vi "TTA_Calibration_Routine.vi"() -> ()   [LabVIEW 2016]
uses:
  TTA_Controls/TTA_Control_Instrument_Cluster.ctl
  TTA_Globals/TTA_Instrument_Cluster.vi
  TTA_Globals/TTA_Global_Working_Directory.vi
  <vilib>/Utility/file.llb/Read Delimited Spreadsheet (string).vi
panel:
  out "Freq Array":T1(array[cluster])
  out "all rows":string[][](array[string])
  in  "Start":bool
  in  "WCS Template":path
  in  "IMT Template":path
  in  "Working Directory":path
  in  "AWS Template":path
  in  "DCS Template":path
  in  "PCS Template":path
  in  "Instrument Cluster":T2
  out "Calibration Status":string
  in  "error in":errorcluster
  out "2D Picture":picture
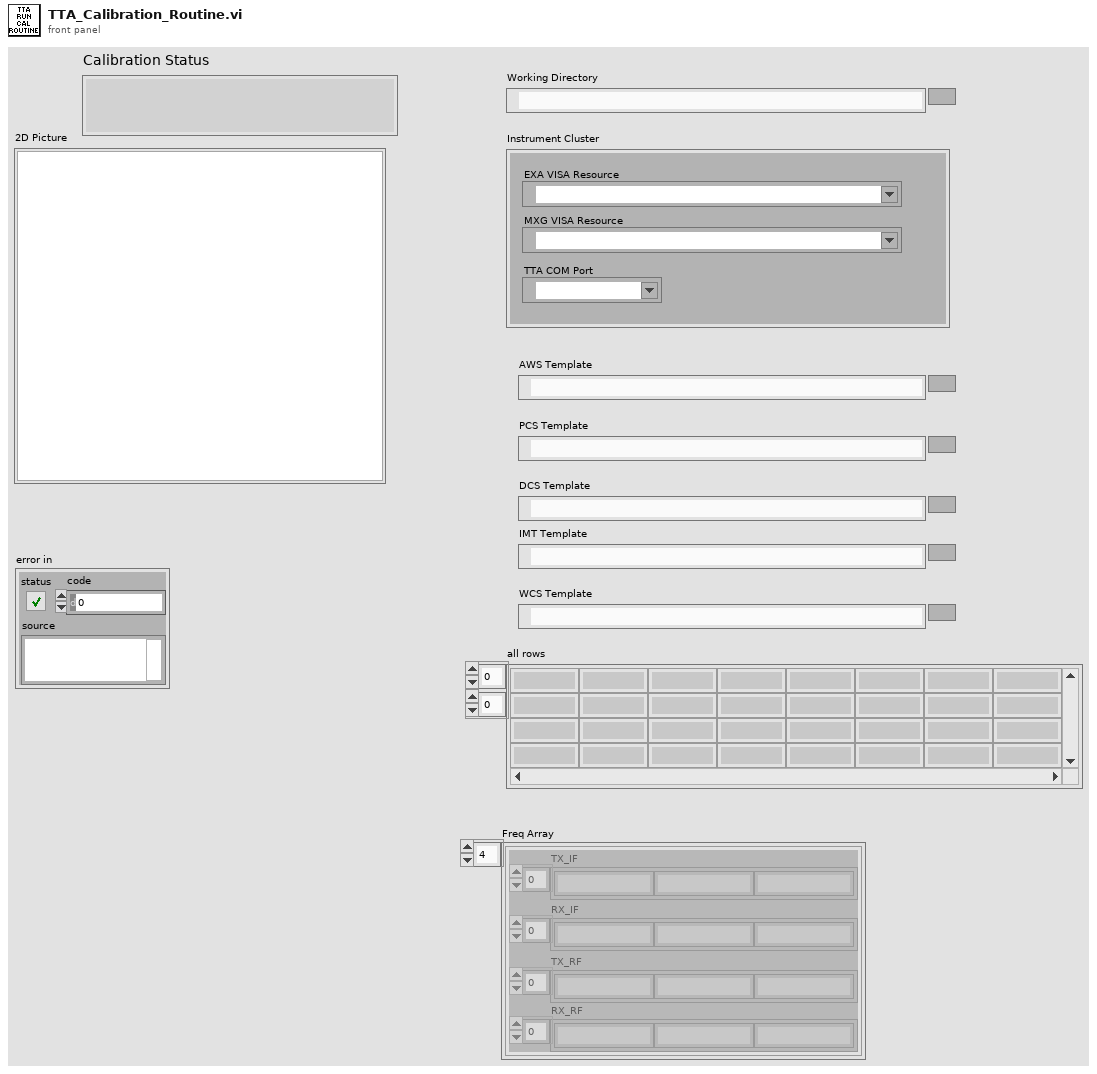
[diagram p1: front panel]
types:
  T1 = cluster{"TX_IF":string[], "RX_IF":string[], "TX_RF":string[], "RX_RF":string[]}[]
  T2 = typedef "TTA_Control_Instrument_Cluster.ctl" = cluster{"EXA VISA Resource":refnum<visa-resource-name>, "MXG VISA Resource":refnum<visa-resource-name>, "TTA COM Port":refnum<visa-resource-name>}
  T3 = cluster{"EXA VISA Resource":refnum<visa-resource-name>, "MXG VISA Resource":refnum<visa-resource-name>, "TTA COM Port":refnum<visa-resource-name>}
  T4 = cluster{"left":i16, "top":i16, "right":i16, "bottom":i16}
  T5 = cluster{"Width":u16, "Style":enum32{"Solid", "Dash", "Dot", "DashDot", "DashDotDot"}}
  T6 = enum16{"TX1", "TX2", "TX3", "TX4", "TXx3", "TXx4", "RX1", "RX2", "RX3", "RX4", "RXx3", "RXx4", "RFCal"}
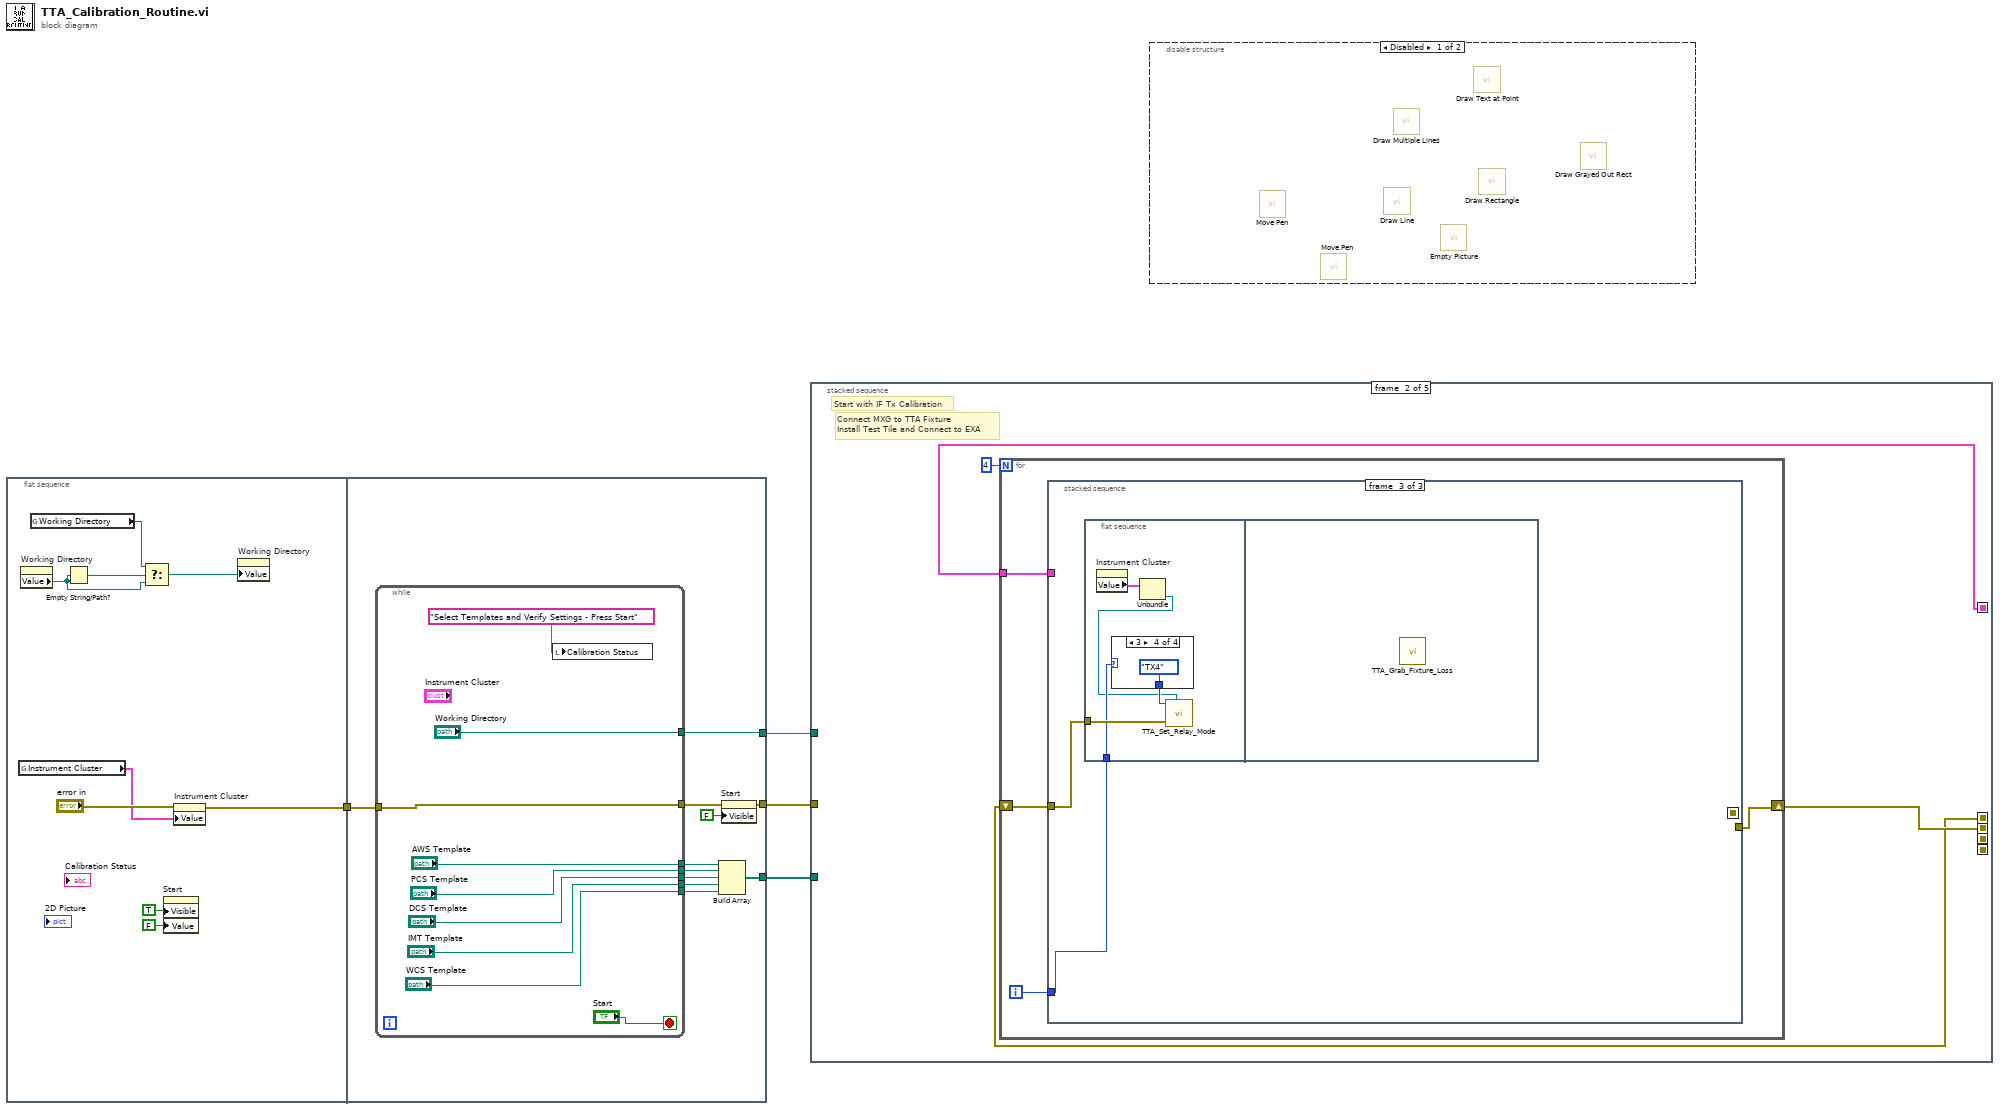
[diagram p0: block diagram]
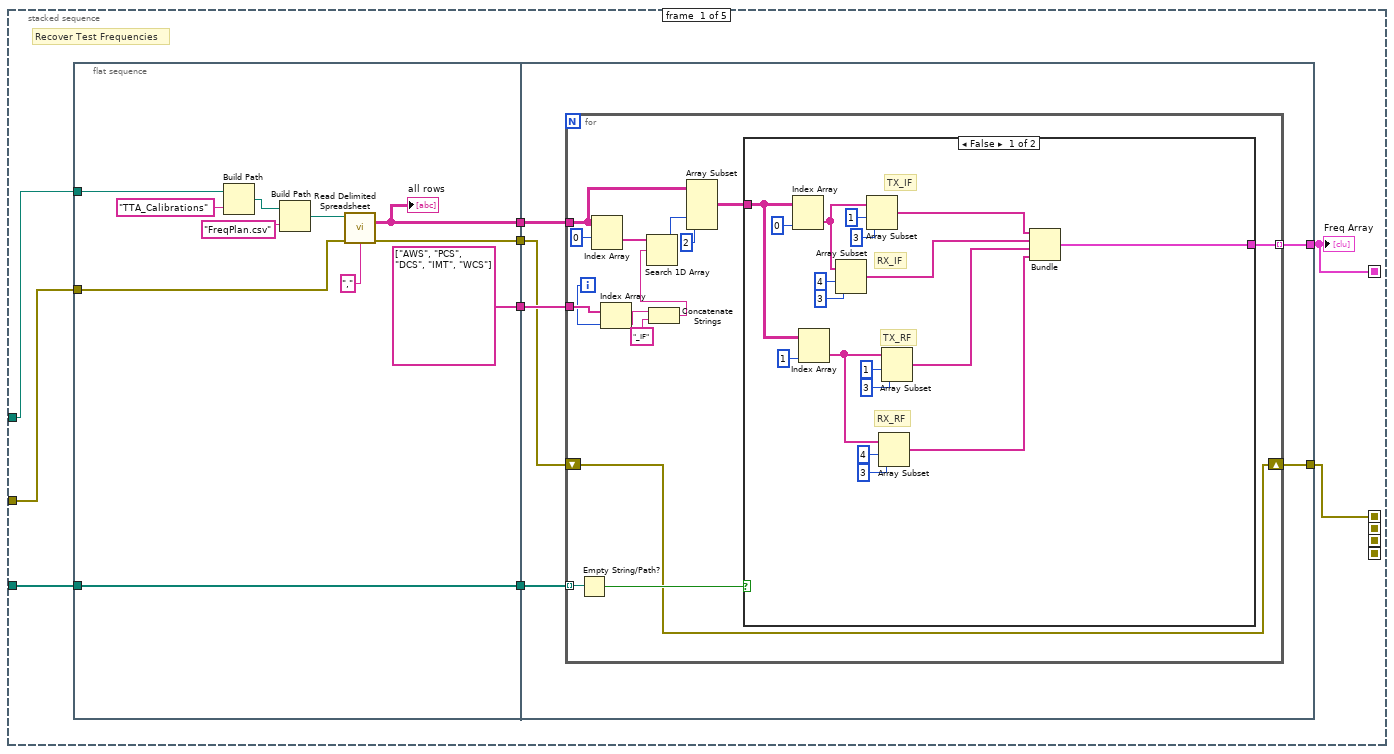
[diagram p3: hidden frame]
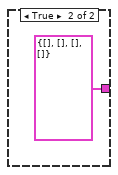
[diagram p4: hidden frame]
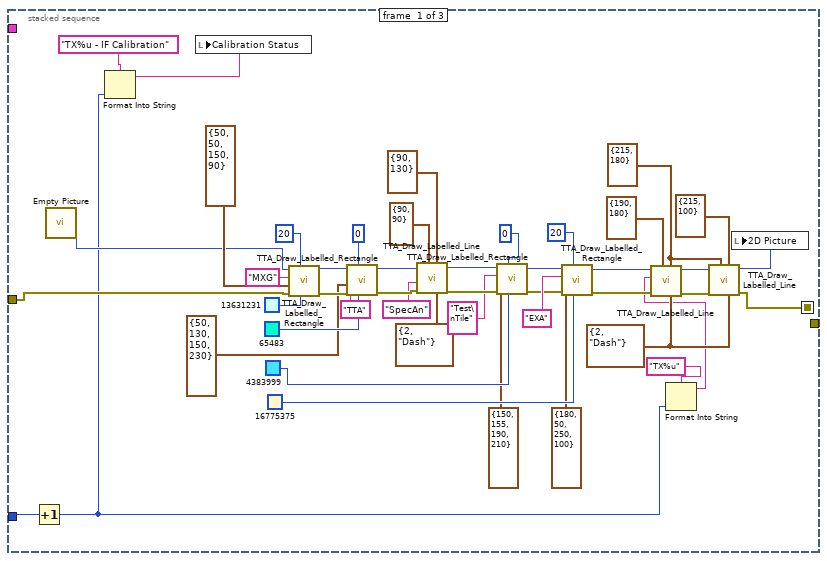
[diagram p5: hidden frame]
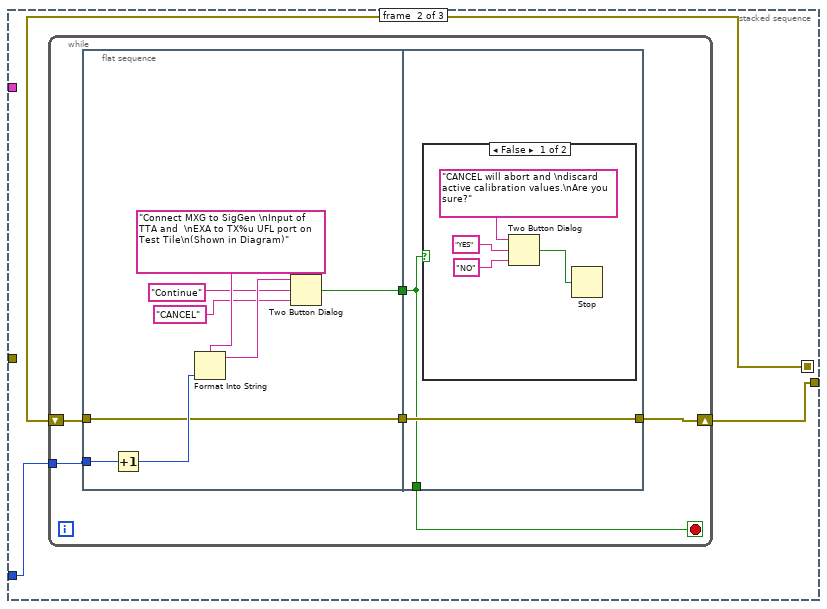
[diagram p6: hidden frame]
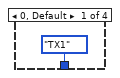
[diagram p8: hidden frame]
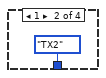
[diagram p9: hidden frame]
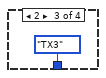
[diagram p10: hidden frame]
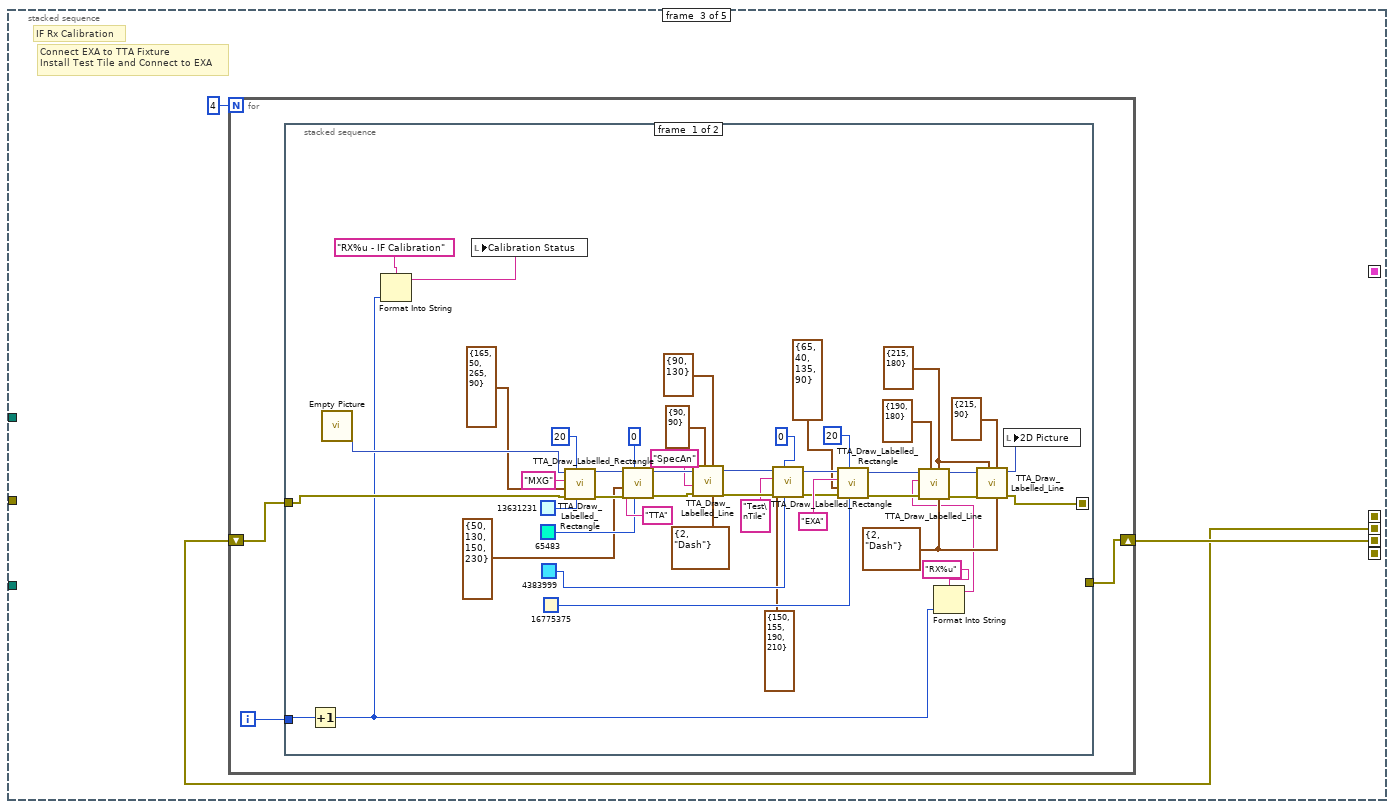
[diagram p11: hidden frame]
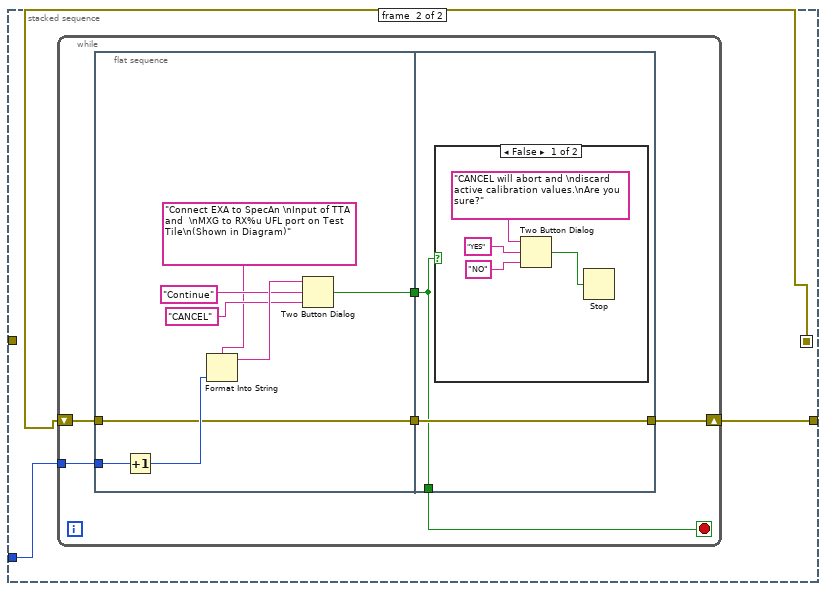
[diagram p12: hidden frame]
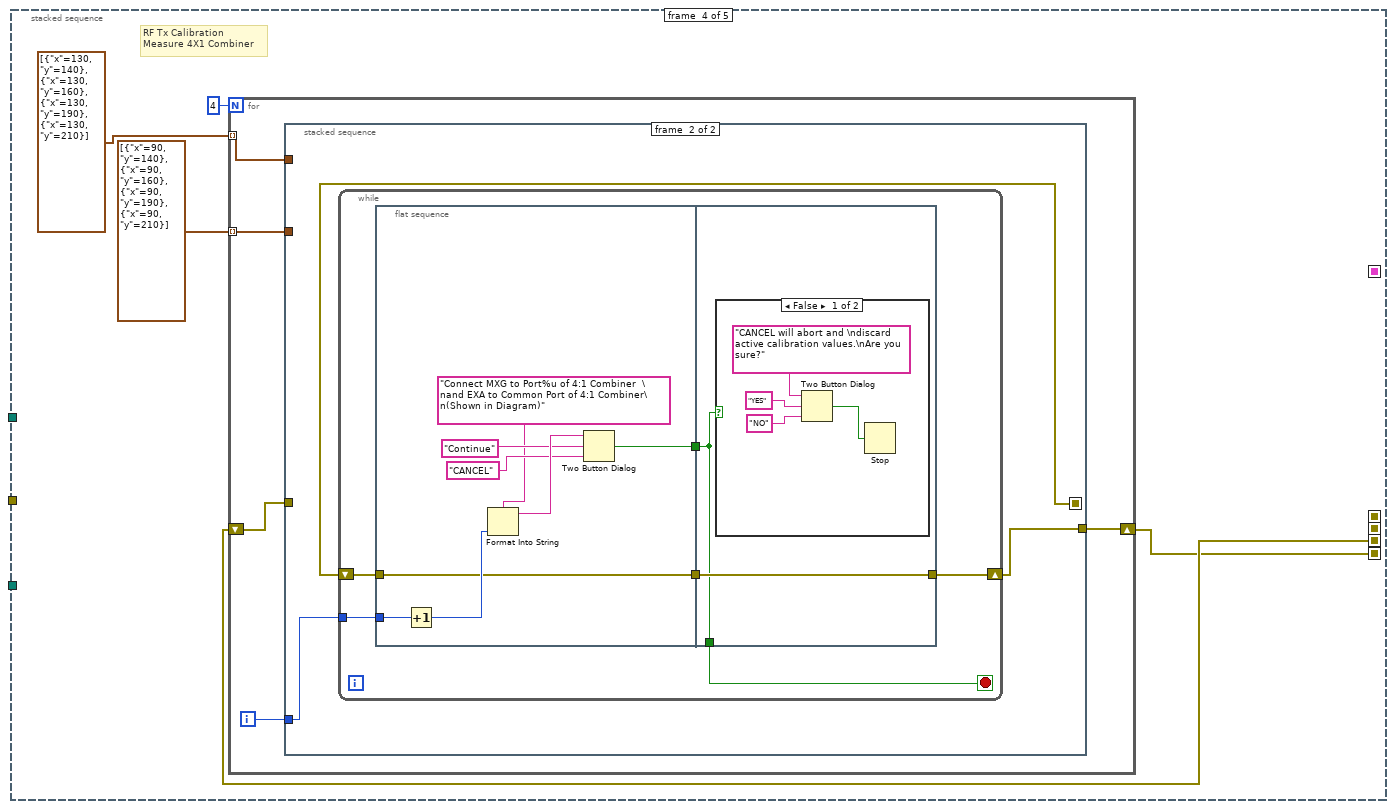
[diagram p14: hidden frame]
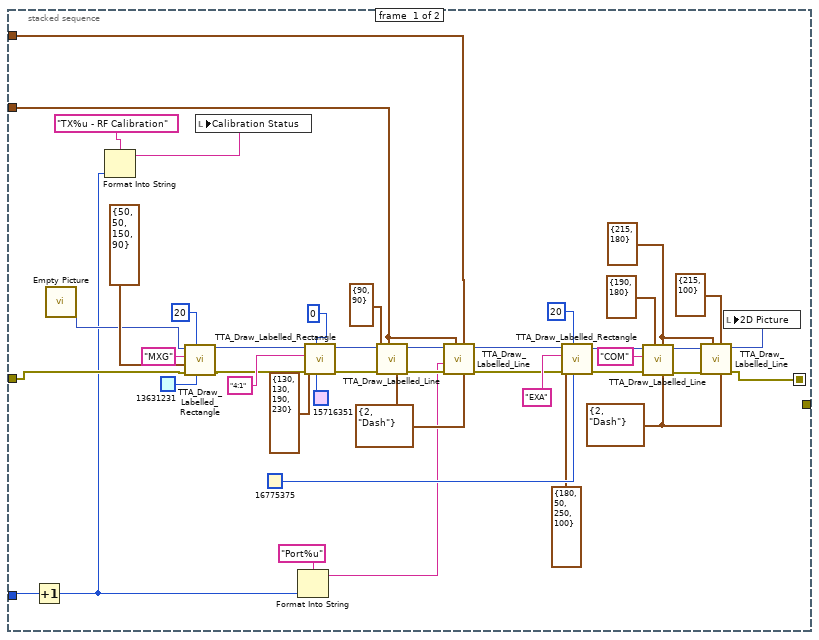
[diagram p15: hidden frame]
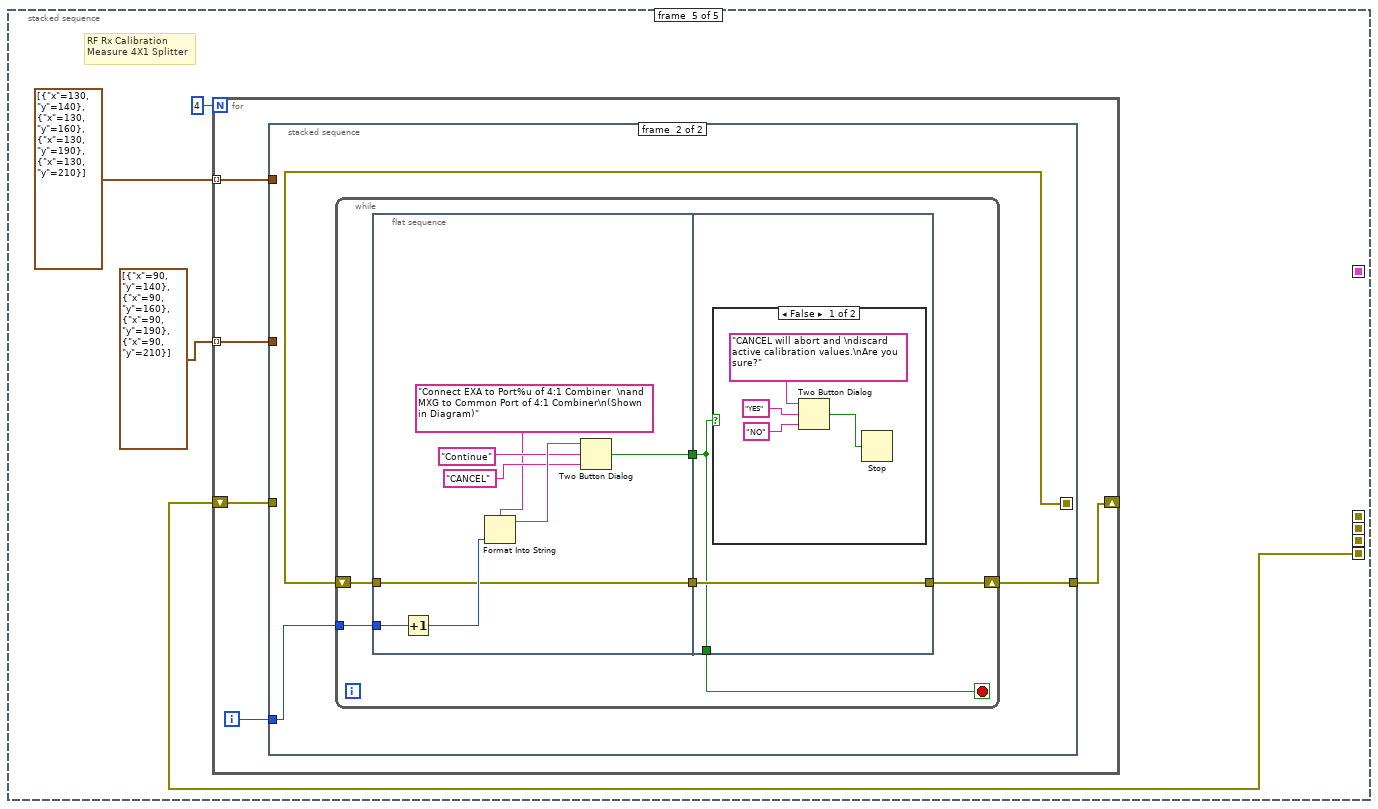
[diagram p17: hidden frame]
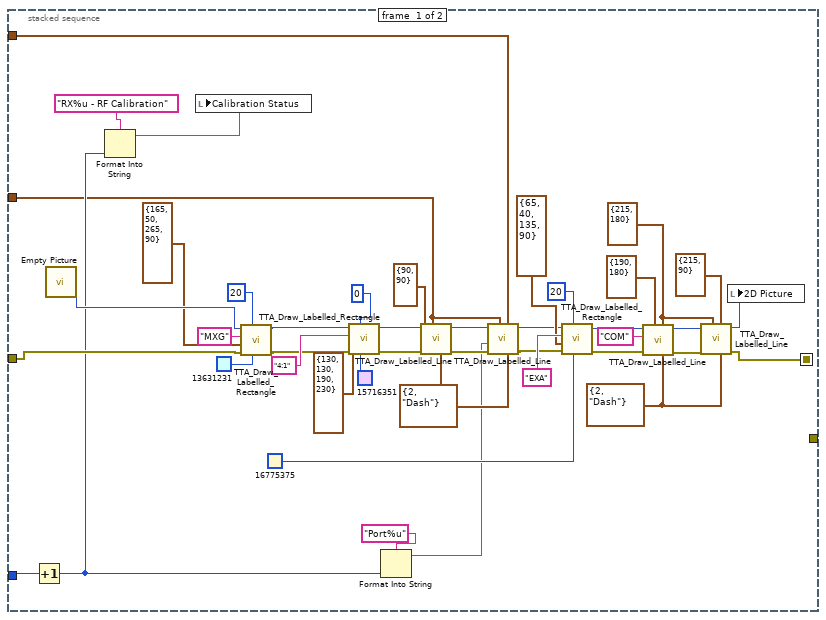
[diagram p18: hidden frame]
diagram:
  n1 = flat-sequence {
    tunnel: [w11] -> w4
    tunnel: w4 -> [w23]
    tunnel: [w21] -> w3
    tunnel: [w20] -> w2
    tunnel: [w14] -> w1
    frame #0 {
      n2 = global read "TTA_Instrument_Cluster.vi" "Instrument Cluster"() -> (w9:T3)
      n3 = property on="Working Directory" class="Path"() -> ("Value"=w6:path)  [unwired: 2 in, 2 out]
      n4 = global read "TTA_Global_Working_Directory.vi" "Working Directory"() -> (w12:path)
      n5 = Empty String/Path?(string/path=w6) -> (empty?=w13:bool)
      n6 = Select(t=w12, s=w13, f=w6) -> (s? t:f=w5:path)
      n7 = property on="Start" class="Bool (strict)"("Visible"=TRUE, "Value"=FALSE ("Start")) -> ()  [unwired: 2 in, 2 out]
      n8 = property on="Instrument Cluster" class="Clust (strict)"(error in="error in", "Value"=w9) -> (error out=w11:errorcluster)  [unwired: 1 in, 1 out]
      n9 = property on="Working Directory" class="Path"("Value"=w5) -> ()  [unwired: 2 in, 2 out]
    }
    frame #1 {
      n10 = while {
        tunnel: w23 -> [w32]
        tunnel: [w32] -> w22
        tunnel: ["Working Directory"] -> w20
        tunnel: ["AWS Template"] -> w19
        tunnel: ["PCS Template"] -> w18
        tunnel: ["DCS Template"] -> w17
        tunnel: ["IMT Template"] -> w16
        tunnel: ["WCS Template"] -> w15
        stop <- "Start" stop-if-true
        n11 = local write "Calibration Status"("Select Templates and Verify Settings - Press Start" ("Calibration Status")) -> ()
      }
      n12 = Build Array(w19, w18, w17, w16, w15) -> (w14:path[])
      n13 = property on="Start" class="Bool (strict)"(error in=w22, "Visible"=FALSE) -> (error out=w21:errorcluster)  [unwired: 1 in, 1 out]
    }
  }
  n14 = stacked-sequence {
    seq-local: [_ w96 _ _ _] -> [_ _ w182 _ _]
    seq-local: [_ _ w183 _ _] -> [_ _ _ w258 _]
    seq-local: [_ _ _ w257 _] -> [_ _ _ _ w333]
    seq-local: [w35 _ _ _ _] -> [_ w94 _ _ _]
    seq-local: [w34 _ _ _ _] -> [_ w95 _ _ _]
    tunnel: w3 -> [w41 _ _ _ _]
    tunnel: w2 -> [w42 _ _ _ _]
    tunnel: w1 -> [w40 _ _ _ _]
    frame #0 {
      # "Recover Test Frequencies"
      n15 = flat-sequence {
        tunnel: w42 -> [w50]
        tunnel: w41 -> [w47]
        tunnel: w40 -> [w46]
        tunnel: [w46] -> w39
        tunnel: [w45] -> w38
        tunnel: [string[] ["AWS", "PCS", "DCS", "IMT", "WCS"]] -> w37
        tunnel: [w43] -> w36
        tunnel: w39 -> [w59]
        tunnel: w38 -> [w58]
        tunnel: w37 -> [w57]
        tunnel: [w56] -> w35
        tunnel: w36 -> [w55]
        tunnel: [w54] -> w34
        frame #0 {
          n16 = Build Path(base path=w50, name or relative path="TTA_Calibrations") -> (appended path=w52:path)
          n17 = Build Path(base path=w52, name or relative path="FreqPlan.csv") -> (appended path=w49:path)
          n18 = call-poly <vilib>:"Read Delimited Spreadsheet.vi"("file path (dialog if empty)"=w49, "error in (no error)"=w47, "delimiter (\\t)"="," ("delimiter (\\t)")) -> ("all rows"=w45:string[][], "error out"=w43:errorcluster)  [unwired: 7 in, 4 out]
          "all rows" <- w45
        }
        frame #1 {
          n19 = for {
            tunnel: w59 -> [w68] mode=indexing
            tunnel: w58 -> [w66]
            tunnel: w57 -> [w74]
            tunnel: [w62] -> w56 mode=indexing
            shift-right: [w61] -> w54
            shift-left: w55 -> [w61]
            i -> [w73]
            n20 = Empty String/Path?(string/path=w68) -> (empty?=w67:bool)
            n21 = Index Array(array=w66, index (row)=0) -> (element=w72:string[])  [unwired: 1 in]
            n22 = Index Array(array=w74, index=w73) -> (element=w71:string)
            n23 = Concatenate Strings(w71, "_IF") -> (w69:string)
            n24 = Search 1D Array(1D array=w72, element=w69) -> (index of element=w65:i32)  [unwired: 1 in]
            n25 = Array Subset(array=w66, index (col)=w65, length (col)=2 ("length")) -> (w63:string[][])  [unwired: 2 in]
            n26 = case shown="False" w67 {
              tunnel: w63 -> [w81 _]
              tunnel: [w90 cluster{string[], string[], string[], string[]} {[], [], [], []}] -> w62
              frame False {
                # "RX_RF"
                # "TX_RF"
                # "RX_IF"
                # "TX_IF"
                n27 = Index Array(array=w81, index (col)=0 ("disabled index (col)")) -> (element=w85:string[])  [unwired: 1 in]
                n28 = Index Array(array=w81, index (col)=1 ("disabled index (col)")) -> (element=w77:string[])  [unwired: 1 in]
                n29 = Array Subset(array=w85, index=4, length=3) -> (w83:string[])
                n30 = Array Subset(array=w85, index=1, length=3) -> (w82:string[])
                n31 = Array Subset(array=w77, index=4, length=3) -> (w91:string[])
                n32 = Array Subset(array=w77, index=1, length=3) -> (w92:string[])
                n33 = Bundle(w82, w83, w92, w91) -> (w90:cluster{string[], string[], string[], string[]})  [unwired: 1 in]
              }
              frame True {
              }
            }
          }
        }
      }
      "Freq Array" <- w35
    }
    frame #1 {
      # "Connect MXG to TTA Fixture\nInstall Test Tile and Connect to EXA"
      # "Start with IF Tx Calibration"
      n34 = for {
        N: 4 -> [_]
        shift-right: [w99] -> w96
        shift-left: w95 -> [w101]
        tunnel: w94 -> [w98]
        i -> [w100]
        n35 = stacked-sequence {
          seq-local: [w107 _ _] -> [_ w149 _]
          tunnel: w101 -> [w111 _ w172]
          tunnel: w100 -> [w109 w150 w171]
          tunnel: [_ w148 _] -> w99
          tunnel: w98 -> [_ _ _]
          frame #0 {
            w118 = T5 {"Width"=2, "Style"=enum."Dash"} ("Line Type")
            w117 = cluster{"x":i16, "y":i16} {"x"=215, "y"=180} ("Start Point")
            n36 = Increment(x=w109) -> (x+1=w103:i32)
            n37 = call "Empty Picture"() -> ("empty picture"=w106:picture)
            n38 = Format Into String(format string="TX%u - IF Calibration" ("Calibration Segment"), w103) -> (resulting string=w104:string)  [unwired: 2 in, 1 out]
            n39 = local write "Calibration Status"(w104) -> ()
            n40 = call "TTA_Draw_Labelled_Rectangle.vi"("color(black)"=u32 13631231, "oval dimension"=i16 20 ("oval height"), "error in"=w111, "Dimensions"=T4 {"left"=50, "top"=50, "right"=150, "bottom"=90} ("MXG"), "Label"="MXG", "picture"=w106) -> ("error out"=w142:errorcluster, "2D Picture\nOut"=w143:picture)  [unwired: 4 in]
            n41 = call "TTA_Draw_Labelled_Rectangle.vi"("color(black)"=u32 65483, "oval dimension"=i16 0, "error in"=w142, "Dimensions"=T4 {"left"=50, "top"=130, "right"=150, "bottom"=230} ("TTA"), "Label"="TTA", "picture"=w143) -> ("error out"=w140:errorcluster, "2D Picture\nOut"=w141:picture)  [unwired: 4 in]
            n42 = call "TTA_Draw_Labelled_Line.vi"("Line Type"=T5 {"Width"=2, "Style"=enum."Dash"}, "End Point"=cluster{"x":i16, "y":i16} {"x"=90, "y"=130} ("Start Point"), "Start Point"=cluster{"x":i16, "y":i16} {"x"=90, "y"=90}, "error in"=w140, "Label\nEnd Point"="SpecAn" ("Label\nEnd Point"), "picture"=w141) -> ("error out"=w133:errorcluster, "2D Picture\nOut"=w134:picture)  [unwired: 4 in]
            n43 = call "TTA_Draw_Labelled_Rectangle.vi"("color(black)"=u32 4383999, "oval dimension"=i16 0, "error in"=w133, "Dimensions"=T4 {"left"=150, "top"=155, "right"=190, "bottom"=210} ("TTile"), "Label"="Test\nTile", "picture"=w134) -> ("error out"=w129:errorcluster, "2D Picture\nOut"=w128:picture)  [unwired: 4 in]
            n44 = call "TTA_Draw_Labelled_Rectangle.vi"("color(black)"=u32 16775375, "oval dimension"=i16 20 ("oval height"), "error in"=w129, "Dimensions"=T4 {"left"=180, "top"=50, "right"=250, "bottom"=100} ("EXA"), "Label"="EXA", "picture"=w128) -> ("error out"=w121:errorcluster, "2D Picture\nOut"=w123:picture)  [unwired: 4 in]
            n45 = Format Into String(format string="TX%u" ("Label\nStart Point"), w103) -> (resulting string=w108:string)  [unwired: 2 in, 1 out]
            n46 = call "TTA_Draw_Labelled_Line.vi"("Line Type"=w118, "End Point"=w117, "Start Point"=cluster{"x":i16, "y":i16} {"x"=190, "y"=180}, "error in"=w121, "Label\nStart Point"=w108, "picture"=w123) -> ("error out"=w120:errorcluster, "2D Picture\nOut"=w119:picture)  [unwired: 4 in]
            n47 = call "TTA_Draw_Labelled_Line.vi"("Line Type"=w118, "End Point"=cluster{"x":i16, "y":i16} {"x"=215, "y"=100} ("Start Point"), "Start Point"=w117, "error in"=w120, "picture"=w119) -> ("error out"=w107:errorcluster, "2D Picture\nOut"=w102:picture)  [unwired: 5 in]
            n48 = local write "2D Picture"(w102) -> ()
          }
          frame #1 {
            n49 = while {
              shift-right: [w154] -> w148
              shift-left: w149 -> [w151]
              tunnel: w150 -> [w152]
              stop <- w153 stop-if-true
              n50 = flat-sequence {
                tunnel: w151 -> [w161]
                tunnel: [w161] -> w156
                tunnel: [w158] -> w155
                tunnel: w152 -> [w157]
                tunnel: [w166] -> w154
                tunnel: w156 -> [w166]
                tunnel: w155 -> [w165]
                tunnel: [w165] -> w153
                frame #0 {
                  n51 = Increment(x=w157) -> (x+1=w164:i32)
                  n52 = Format Into String(format string="Connect MXG to SigGen \nInput of TTA and  \nEXA to TX%u UFL port on Test Tile\n(Shown in Diagram)" ("message"), w164) -> (resulting string=w162:string)  [unwired: 2 in, 1 out]
                  n53 = Two Button Dialog(message=w162, 1:"CANCEL" ("button name (\"OK\")"), 2:"Continue" ("button name (\"OK\")")) -> (T button?=w158:bool)
                }
                frame #1 {
                  n54 = case shown="False" w165 {
                    frame False {
                      n55 = Two Button Dialog(message="CANCEL will abort and \ndiscard active calibration values.\nAre you sure?", 1:"NO" ("F button name (\"Cancel\")"), 2:"YES" ("T button name (\"OK\")")) -> (T button?=w167:bool)
                      n56 = Stop(stop? (T)=w167) -> ()
                    }
                    frame True {
                    }
                  }
                }
              }
            }
          }
          frame #2 {
            n57 = flat-sequence {
              tunnel: w172 -> [w177]
              tunnel: w171 -> [w176]
              frame #0 {
                n58 = property on="Instrument Cluster" class="Clust (strict)"() -> ("Value"=w174:T2)  [unwired: 2 in, 2 out]
                n59 = case shown="3" w176 {
                  tunnel: [T6."TX1" ("Mode") T6."TX2" ("Mode") T6."TX3" ("Mode") T6."TX4" ("Mode")] -> w175
                  frame 0, Default {
                  }
                  frame 1 {
                  }
                  frame 2 {
                  }
                  frame 3 {
                  }
                }
                n60 = Unbundle(w174) -> ("TTA COM Port"=w173:refnum<visa-resource-name>)  [unwired: 2 out]
                n61 = call "TTA_Set_Relay_Mode.vi"("TTA COM Port"=w173, "error in"=w177, "Mode"=w175) -> ()  [unwired: 8 in, 1 out]
              }
              frame #1 {
                n62 = call "TTA_Grab_Fixture_Loss.vi"() -> ()  [unwired: 16 in]
              }
            }
          }
        }
      }
    }
    frame #2 {
      # "Connect EXA to TTA Fixture\nInstall Test Tile and Connect to EXA"
      # "IF Rx Calibration"
      n63 = for {
        N: 4 -> [_]
        shift-right: [w185] -> w183
        shift-left: w182 -> [w187]
        i -> [w186]
        n64 = stacked-sequence {
          seq-local: [w195 _] -> [_ w236]
          tunnel: w187 -> [w199 _]
          tunnel: w186 -> [w197 w235]
          tunnel: [_ w234] -> w185
          frame #0 {
            w204 = T5 {"Width"=2, "Style"=enum."Dash"} ("Line Type")
            w203 = cluster{"x":i16, "y":i16} {"x"=215, "y"=180} ("Start Point")
            n65 = Increment(x=w197) -> (x+1=w191:i32)
            n66 = call "Empty Picture"() -> ("empty picture"=w194:picture)
            n67 = Format Into String(format string="RX%u - IF Calibration" ("Calibration Segment"), w191) -> (resulting string=w192:string)  [unwired: 2 in, 1 out]
            n68 = local write "Calibration Status"(w192) -> ()
            n69 = call "TTA_Draw_Labelled_Rectangle.vi"("color(black)"=u32 13631231, "oval dimension"=i16 20 ("oval height"), "error in"=w199, "Dimensions"=T4 {"left"=165, "top"=50, "right"=265, "bottom"=90} ("EXA"), "Label"="MXG", "picture"=w194) -> ("error out"=w228:errorcluster, "2D Picture\nOut"=w229:picture)  [unwired: 4 in]
            n70 = call "TTA_Draw_Labelled_Rectangle.vi"("color(black)"=u32 65483, "oval dimension"=i16 0, "error in"=w228, "Dimensions"=T4 {"left"=50, "top"=130, "right"=150, "bottom"=230} ("TTA"), "Label"="TTA", "picture"=w229) -> ("error out"=w226:errorcluster, "2D Picture\nOut"=w227:picture)  [unwired: 4 in]
            n71 = call "TTA_Draw_Labelled_Line.vi"("Line Type"=T5 {"Width"=2, "Style"=enum."Dash"}, "End Point"=cluster{"x":i16, "y":i16} {"x"=90, "y"=130} ("Start Point"), "Start Point"=cluster{"x":i16, "y":i16} {"x"=90, "y"=90}, "error in"=w226, "Label\nEnd Point"="SpecAn" ("Label\nEnd Point"), "picture"=w227) -> ("error out"=w219:errorcluster, "2D Picture\nOut"=w220:picture)  [unwired: 4 in]
            n72 = call "TTA_Draw_Labelled_Rectangle.vi"("color(black)"=u32 4383999, "oval dimension"=i16 0, "error in"=w219, "Dimensions"=T4 {"left"=150, "top"=155, "right"=190, "bottom"=210} ("TTile"), "Label"="Test\nTile", "picture"=w220) -> ("error out"=w215:errorcluster, "2D Picture\nOut"=w214:picture)  [unwired: 4 in]
            n73 = call "TTA_Draw_Labelled_Rectangle.vi"("color(black)"=u32 16775375, "oval dimension"=i16 20 ("oval height"), "error in"=w215, "Dimensions"=T4 {"left"=65, "top"=40, "right"=135, "bottom"=90} ("MXG"), "Label"="EXA", "picture"=w214) -> ("error out"=w207:errorcluster, "2D Picture\nOut"=w209:picture)  [unwired: 4 in]
            n74 = Format Into String(format string="RX%u" ("Label\nStart Point"), w191) -> (resulting string=w196:string)  [unwired: 2 in, 1 out]
            n75 = call "TTA_Draw_Labelled_Line.vi"("Line Type"=w204, "End Point"=w203, "Start Point"=cluster{"x":i16, "y":i16} {"x"=190, "y"=180}, "error in"=w207, "Label\nStart Point"=w196, "picture"=w209) -> ("error out"=w206:errorcluster, "2D Picture\nOut"=w205:picture)  [unwired: 4 in]
            n76 = call "TTA_Draw_Labelled_Line.vi"("Line Type"=w204, "End Point"=cluster{"x":i16, "y":i16} {"x"=215, "y"=90} ("Start Point"), "Start Point"=w203, "error in"=w206, "picture"=w205) -> ("error out"=w195:errorcluster, "2D Picture\nOut"=w190:picture)  [unwired: 5 in]
            n77 = local write "2D Picture"(w190) -> ()
          }
          frame #1 {
            n78 = while {
              shift-right: [w239] -> w234
              shift-left: w236 -> [w240]
              tunnel: w235 -> [w237]
              stop <- w238 stop-if-true
              n79 = flat-sequence {
                tunnel: w240 -> [w248]
                tunnel: [w248] -> w242
                tunnel: [w245] -> w241
                tunnel: w237 -> [w243]
                tunnel: [w252] -> w239
                tunnel: w242 -> [w252]
                tunnel: w241 -> [w251]
                tunnel: [w251] -> w238
                frame #0 {
                  n80 = Increment(x=w243) -> (x+1=w250:i32)
                  n81 = Format Into String(format string="Connect EXA to SpecAn \nInput of TTA and  \nMXG to RX%u UFL port on Test Tile\n(Shown in Diagram)" ("message"), w250) -> (resulting string=w249:string)  [unwired: 2 in, 1 out]
                  n82 = Two Button Dialog(message=w249, 1:"CANCEL" ("button name (\"OK\")"), 2:"Continue" ("button name (\"OK\")")) -> (T button?=w245:bool)
                }
                frame #1 {
                  n83 = case shown="False" w251 {
                    frame False {
                      n84 = Two Button Dialog(message="CANCEL will abort and \ndiscard active calibration values.\nAre you sure?", 1:"NO" ("F button name (\"Cancel\")"), 2:"YES" ("T button name (\"OK\")")) -> (T button?=w253:bool)
                      n85 = Stop(stop? (T)=w253) -> ()
                    }
                    frame True {
                    }
                  }
                }
              }
            }
          }
        }
      }
    }
    frame #3 {
      # "RF Tx Calibration\nMeasure 4X1 Combiner"
      n86 = for {
        N: 4 -> [_]
        shift-right: [w264] -> w257
        shift-left: w258 -> [w266]
        tunnel: cluster{"x":i16, "y":i16}[] [{"x"=90, "y"=140}, {"x"=90, "y"=160}, {"x"=90, "y"=190}, {"x"=90, "y"=210}] -> [w263] mode=indexing
        tunnel: cluster{"x":i16, "y":i16}[] [{"x"=130, "y"=140}, {"x"=130, "y"=160}, {"x"=130, "y"=190}, {"x"=130, "y"=210}] -> [w262] mode=indexing
        i -> [w265]
        n87 = stacked-sequence {
          seq-local: [w289 _] -> [_ w311]
          tunnel: w266 -> [w292 _]
          tunnel: w265 -> [w290 w310]
          tunnel: [_ w312] -> w264
          tunnel: w263 -> [w268 _]
          tunnel: w262 -> [w267 _]
          frame #0 {
            w297 = T5 {"Width"=2, "Style"=enum."Dash"} ("Line Type")
            w296 = cluster{"x":i16, "y":i16} {"x"=215, "y"=180} ("Start Point")
            w275 = T5 {"Width"=2, "Style"=enum."Dash"} ("Line Type")
            n88 = Increment(x=w290) -> (x+1=w285:i32)
            n89 = call "Empty Picture"() -> ("empty picture"=w288:picture)
            n90 = Format Into String(format string="TX%u - RF Calibration" ("Calibration Segment"), w285) -> (resulting string=w286:string)  [unwired: 2 in, 1 out]
            n91 = call "TTA_Draw_Labelled_Rectangle.vi"("color(black)"=u32 13631231, "oval dimension"=i16 20 ("oval height"), "error in"=w292, "Dimensions"=T4 {"left"=50, "top"=50, "right"=150, "bottom"=90} ("MXG"), "Label"="MXG", "picture"=w288) -> ("error out"=w277:errorcluster, "2D Picture\nOut"=w279:picture)  [unwired: 4 in]
            n92 = local write "Calibration Status"(w286) -> ()
            n93 = Format Into String(format string="Port%u" ("Label\nStart Point"), w285) -> (resulting string=w270:string)  [unwired: 2 in, 1 out]
            n94 = call "TTA_Draw_Labelled_Rectangle.vi"("color(black)"=u32 15716351, "oval dimension"=i16 0, "error in"=w277, "Dimensions"=T4 {"left"=130, "top"=130, "right"=190, "bottom"=230} ("TTile"), "Label"="4:1", "picture"=w279) -> ("error out"=w276:errorcluster, "2D Picture\nOut"=w278:picture)  [unwired: 4 in]
            n95 = call "TTA_Draw_Labelled_Line.vi"("Line Type"=w275, "End Point"=w268, "Start Point"=cluster{"x":i16, "y":i16} {"x"=90, "y"=90}, "error in"=w276, "picture"=w278) -> ("error out"=w274:errorcluster, "2D Picture\nOut"=w273:picture)  [unwired: 5 in]
            n96 = call "TTA_Draw_Labelled_Line.vi"("Line Type"=w275, "End Point"=w267, "Start Point"=w268, "error in"=w274, "Label\nEnd Point"=w270, "picture"=w273) -> ("error out"=w271:errorcluster, "2D Picture\nOut"=w272:picture)  [unwired: 4 in]
            n97 = call "TTA_Draw_Labelled_Rectangle.vi"("color(black)"=u32 16775375, "oval dimension"=i16 20 ("oval height"), "error in"=w271, "Dimensions"=T4 {"left"=180, "top"=50, "right"=250, "bottom"=100} ("EXA"), "Label"="EXA", "picture"=w272) -> ("error out"=w300:errorcluster, "2D Picture\nOut"=w302:picture)  [unwired: 4 in]
            n98 = call "TTA_Draw_Labelled_Line.vi"("Line Type"=w297, "End Point"=w296, "Start Point"=cluster{"x":i16, "y":i16} {"x"=190, "y"=180}, "error in"=w300, "Label\nStart Point"="COM" ("Label\nStart Point"), "picture"=w302) -> ("error out"=w299:errorcluster, "2D Picture\nOut"=w298:picture)  [unwired: 4 in]
            n99 = call "TTA_Draw_Labelled_Line.vi"("Line Type"=w297, "End Point"=cluster{"x":i16, "y":i16} {"x"=215, "y"=100} ("Start Point"), "Start Point"=w296, "error in"=w299, "picture"=w298) -> ("error out"=w289:errorcluster, "2D Picture\nOut"=w284:picture)  [unwired: 5 in]
            n100 = local write "2D Picture"(w284) -> ()
          }
          frame #1 {
            n101 = while {
              shift-right: [w315] -> w312
              shift-left: w311 -> [w316]
              tunnel: w310 -> [w313]
              stop <- w314 stop-if-true
              n102 = flat-sequence {
                tunnel: w316 -> [w324]
                tunnel: [w324] -> w318
                tunnel: [w321] -> w317
                tunnel: w313 -> [w319]
                tunnel: [w328] -> w315
                tunnel: w318 -> [w328]
                tunnel: w317 -> [w327]
                tunnel: [w327] -> w314
                frame #0 {
                  n103 = Increment(x=w319) -> (x+1=w326:i32)
                  n104 = Format Into String(format string="Connect MXG to Port%u of 4:1 Combiner  \nand EXA to Common Port of 4:1 Combiner\n(Shown in Diagram)" ("message"), w326) -> (resulting string=w325:string)  [unwired: 2 in, 1 out]
                  n105 = Two Button Dialog(message=w325, 1:"CANCEL" ("button name (\"OK\")"), 2:"Continue" ("button name (\"OK\")")) -> (T button?=w321:bool)
                }
                frame #1 {
                  n106 = case shown="False" w327 {
                    frame False {
                      n107 = Two Button Dialog(message="CANCEL will abort and \ndiscard active calibration values.\nAre you sure?", 1:"NO" ("F button name (\"Cancel\")"), 2:"YES" ("T button name (\"OK\")")) -> (T button?=w329:bool)
                      n108 = Stop(stop? (T)=w329) -> ()
                    }
                    frame True {
                    }
                  }
                }
              }
            }
          }
        }
      }
    }
    frame #4 {
      # "RF Rx Calibration\nMeasure 4X1 Splitter"
      n109 = for {
        N: 4 -> [_]
        shift-right: [w339] -> _
        shift-left: w333 -> [w341]
        tunnel: cluster{"x":i16, "y":i16}[] [{"x"=90, "y"=140}, {"x"=90, "y"=160}, {"x"=90, "y"=190}, {"x"=90, "y"=210}] -> [w338] mode=indexing
        tunnel: cluster{"x":i16, "y":i16}[] [{"x"=130, "y"=140}, {"x"=130, "y"=160}, {"x"=130, "y"=190}, {"x"=130, "y"=210}] -> [w337] mode=indexing
        i -> [w340]
        n110 = stacked-sequence {
          seq-local: [w367 _] -> [_ w385]
          tunnel: w341 -> [w370 _]
          tunnel: w340 -> [w368 w386]
          tunnel: [_ w387] -> w339
          tunnel: w338 -> [w347 _]
          tunnel: w337 -> [w346 _]
          frame #0 {
            w352 = T5 {"Width"=2, "Style"=enum."Dash"} ("Line Type")
            w373 = T5 {"Width"=2, "Style"=enum."Dash"} ("Line Type")
            w372 = cluster{"x":i16, "y":i16} {"x"=215, "y"=180} ("Start Point")
            n111 = Increment(x=w368) -> (x+1=w363:i32)
            n112 = call "Empty Picture"() -> ("empty picture"=w366:picture)
            n113 = Format Into String(format string="RX%u - RF Calibration" ("Calibration Segment"), w363) -> (resulting string=w364:string)  [unwired: 2 in, 1 out]
            n114 = local write "Calibration Status"(w364) -> ()
            n115 = call "TTA_Draw_Labelled_Rectangle.vi"("color(black)"=u32 13631231, "oval dimension"=i16 20 ("oval height"), "error in"=w370, "Dimensions"=T4 {"left"=165, "top"=50, "right"=265, "bottom"=90} ("EXA"), "Label"="MXG", "picture"=w366) -> ("error out"=w348:errorcluster, "2D Picture\nOut"=w349:picture)  [unwired: 4 in]
            n116 = call "TTA_Draw_Labelled_Rectangle.vi"("color(black)"=u32 15716351, "oval dimension"=i16 0, "error in"=w348, "Dimensions"=T4 {"left"=130, "top"=130, "right"=190, "bottom"=230} ("TTile"), "Label"="4:1", "picture"=w349) -> ("error out"=w353:errorcluster, "2D Picture\nOut"=w354:picture)  [unwired: 4 in]
            n117 = Format Into String(format string="Port%u" ("Label\nStart Point"), w363) -> (resulting string=w343:string)  [unwired: 2 in, 1 out]
            n118 = call "TTA_Draw_Labelled_Line.vi"("Line Type"=w352, "End Point"=w347, "Start Point"=cluster{"x":i16, "y":i16} {"x"=90, "y"=90}, "error in"=w353, "picture"=w354) -> ("error out"=w351:errorcluster, "2D Picture\nOut"=w350:picture)  [unwired: 5 in]
            n119 = call "TTA_Draw_Labelled_Line.vi"("Line Type"=w352, "End Point"=w346, "Start Point"=w347, "error in"=w351, "Label\nEnd Point"=w343, "picture"=w350) -> ("error out"=w344:errorcluster, "2D Picture\nOut"=w345:picture)  [unwired: 4 in]
            n120 = call "TTA_Draw_Labelled_Rectangle.vi"("color(black)"=u32 16775375, "oval dimension"=i16 20 ("oval height"), "error in"=w344, "Dimensions"=T4 {"left"=65, "top"=40, "right"=135, "bottom"=90} ("MXG"), "Label"="EXA", "picture"=w345) -> ("error out"=w376:errorcluster, "2D Picture\nOut"=w378:picture)  [unwired: 4 in]
            n121 = call "TTA_Draw_Labelled_Line.vi"("Line Type"=w373, "End Point"=w372, "Start Point"=cluster{"x":i16, "y":i16} {"x"=190, "y"=180}, "error in"=w376, "Label\nStart Point"="COM" ("Label\nStart Point"), "picture"=w378) -> ("error out"=w375:errorcluster, "2D Picture\nOut"=w374:picture)  [unwired: 4 in]
            n122 = call "TTA_Draw_Labelled_Line.vi"("Line Type"=w373, "End Point"=cluster{"x":i16, "y":i16} {"x"=215, "y"=90} ("Start Point"), "Start Point"=w372, "error in"=w375, "picture"=w374) -> ("error out"=w367:errorcluster, "2D Picture\nOut"=w362:picture)  [unwired: 5 in]
            n123 = local write "2D Picture"(w362) -> ()
          }
          frame #1 {
            n124 = while {
              shift-right: [w390] -> w387
              shift-left: w385 -> [w391]
              tunnel: w386 -> [w388]
              stop <- w389 stop-if-true
              n125 = flat-sequence {
                tunnel: w391 -> [w399]
                tunnel: [w399] -> w393
                tunnel: [w396] -> w392
                tunnel: w388 -> [w394]
                tunnel: [w403] -> w390
                tunnel: w393 -> [w403]
                tunnel: w392 -> [w402]
                tunnel: [w402] -> w389
                frame #0 {
                  n126 = Increment(x=w394) -> (x+1=w401:i32)
                  n127 = Format Into String(format string="Connect EXA to Port%u of 4:1 Combiner  \nand MXG to Common Port of 4:1 Combiner\n(Shown in Diagram)" ("message"), w401) -> (resulting string=w400:string)  [unwired: 2 in, 1 out]
                  n128 = Two Button Dialog(message=w400, 1:"CANCEL" ("button name (\"OK\")"), 2:"Continue" ("button name (\"OK\")")) -> (T button?=w396:bool)
                }
                frame #1 {
                  n129 = case shown="False" w402 {
                    frame False {
                      n130 = Two Button Dialog(message="CANCEL will abort and \ndiscard active calibration values.\nAre you sure?", 1:"NO" ("F button name (\"Cancel\")"), 2:"YES" ("T button name (\"OK\")")) -> (T button?=w404:bool)
                      n131 = Stop(stop? (T)=w404) -> ()
                    }
                    frame True {
                    }
                  }
                }
              }
            }
          }
        }
      }
    }
  }
  n132 = disable-structure shown="Disabled" {
    frame Disabled {
      n133 = call <vilib>:"Move Pen.vi"() -> ()  [unwired: 5 in, 1 out]
      n134 = call <vilib>:"Move Pen.vi"() -> ()  [unwired: 5 in, 1 out]
      n135 = call <vilib>:"Draw Line.vi"() -> ()  [unwired: 9 in, 1 out]
      n136 = call <vilib>:"Draw Multiple Lines.vi"() -> ()  [unwired: 9 in, 1 out]
      n137 = call "Empty Picture"() -> ()  [unwired: 1 out]
      n138 = call <vilib>:"Draw Text at Point.vi"() -> ()  [unwired: 10 in, 2 out]
      n139 = call <vilib>:"Draw Rectangle.vi"() -> ()  [unwired: 9 in, 1 out]
      n140 = call <vilib>:"Draw Grayed Out Rect.vi"() -> ()  [unwired: 5 in, 1 out]
    }
    frame Enabled {
    }
  }
